vi "player.vi"() -> ()   [LabVIEW 2022 SP3]
uses:
  <vilib>/DAQmx/write.llb/DAQmx Write (Digital 1D Bool 1Chan 1Samp).vi
  <vilib>/DAQmx/create/channels.llb/DAQmx Create Channel (DO-Digital Output).vi
  <vilib>/Utility/file.llb/Read Delimited Spreadsheet (DBL).vi
  <vilib>/DAQmx/miscellaneous.llb/DAQmx Fill In Error Info.vi
panel:
  in  "Speed*X(If you want to play X times faster, enter X)":dbl=1.0
  in  "Backwards Mode (Forwards moves the light left to right, top to bottom)":bool
  in  "Choose LED Array (leftmost LED=top switch, rightmost LED=bottom switch":bool[](array[boolean])=[TRUE, FALSE, FALSE, FALSE, FALSE, FALSE, FALSE, FALSE]
  out "Numeric 3":dbl
  out "Numeric 2":dbl
  out "Last Wait":dbl
  out "Wait Times":dbl[](array[numeric])
  out "LEDs":bool[](array[boolean])
  out "error out":errorcluster
  in  "stop":bool
  # "LED Player! Play your own Christmas pattern!"
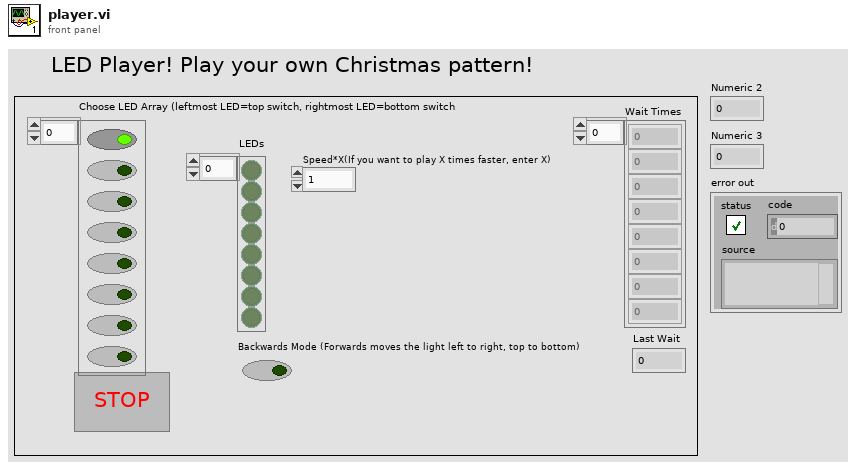
[diagram p1: front panel]
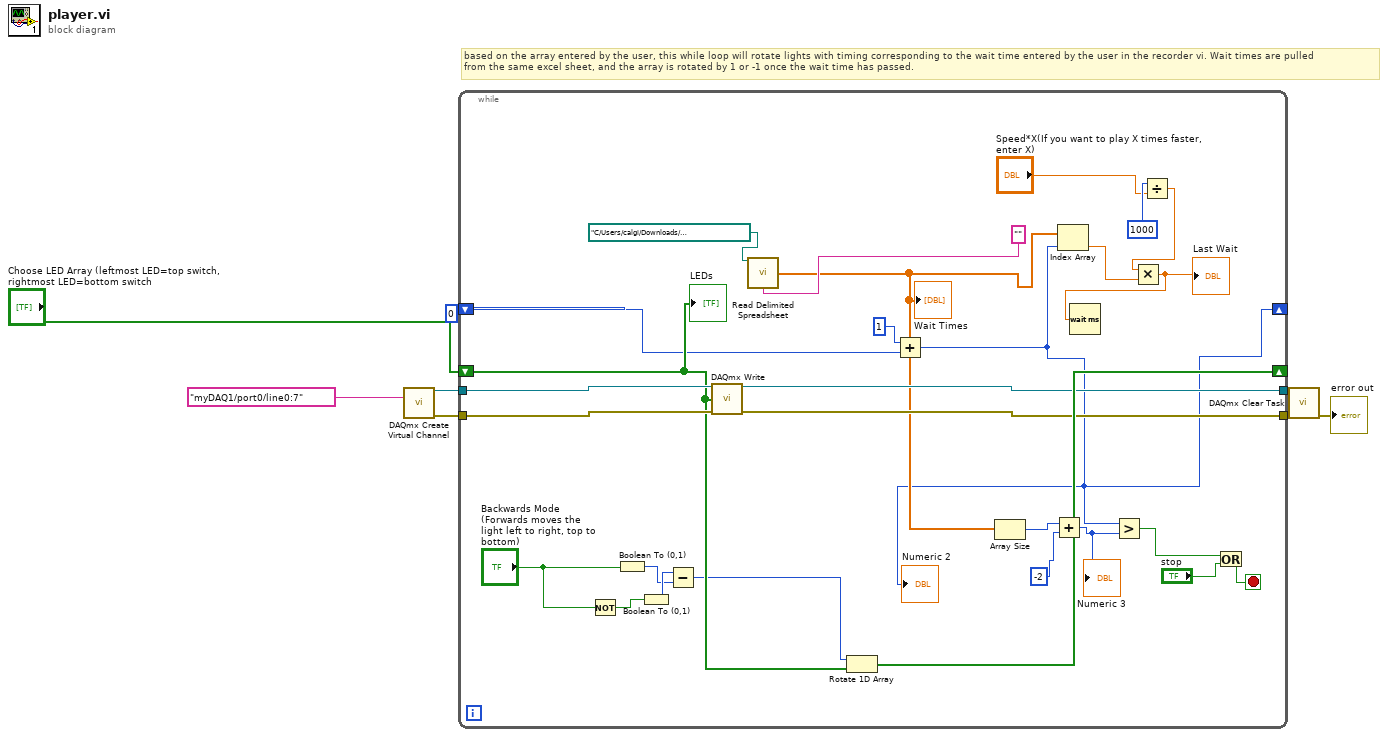
[diagram p0: block diagram]
diagram:
  # "based on the array entered by the user, this while loop will rotate lights with timing corresponding to the wait time entered by the user in the recorder vi. Wait times are pulled\nfrom the same excel sheet, and the array is rotated by 1 or -1 once the wait time has passed."
  n1 = call-poly <vilib>:"DAQmx Create Virtual Channel.vi"("lines"=tag "myDAQ1/port0/line0:7") -> ("task out"=w7:refnum<k21>, "error out"=w6:errorcluster)  [unwired: 13 in]
  n2 = while {
    shift-right: [w36] -> _
    shift-left: "Choose LED Array (leftmost LED=top switch, rightmost LED=bottom switch" -> [w31]
    tunnel: w7 -> [w35]
    tunnel: w6 -> [w34]
    tunnel: [w33] -> w5
    tunnel: [w32] -> w4
    shift-right: [w19] -> _
    shift-left: 0 -> [w28]
    stop <- w20 stop-if-true
    n3 = Not(x="Backwards Mode (Forwards moves the light left to right, top to bottom)") -> (.not. x?=w17:bool)
    n4 = Boolean To (0,1)(Boolean="Backwards Mode (Forwards moves the light left to right, top to bottom)") -> (0, 1=w14:i16)
    n5 = Boolean To (0,1)(Boolean=w17) -> (0, 1=w15:i16)
    n6 = Subtract(x=w15, y=w14) -> (x-y=w13:i16)
    n7 = call-poly <vilib>:"DAQmx Write.vi"("task/channels in"=w35, "data"=w31, "error in"=w34) -> ("task out"=w33:refnum<k21>, "error out"=w32:errorcluster)  [unwired: 10 in, 1 out]
    n8 = call-poly <vilib>:"Read Delimited Spreadsheet.vi"("file path (dialog if empty)"=path "C:/Users/calgi/Downloads/keyboardpatternBeta.csv", "delimiter (\\t)"="") -> ("first row"=w25:dbl[])  [unwired: 8 in, 5 out]
    "Wait Times" <- w25
    n9 = Rotate 1D Array(1:w31, 2:w13) -> (0:w36:bool[])
    n10 = Add(x=1, y=w28) -> (x+y=w19:i32)
    "Numeric 2" <- w19
    n11 = Array Size(array=w25) -> (size(s)=w24:i32)
    n12 = Add(x=w24, y=-2) -> (x+y=w18:i32)
    "Numeric 3" <- w18
    n13 = Index Array(array=w25, index=w19) -> (element=w30:dbl)
    n14 = Greater?(x=w19, y=w18) -> (0:w21:bool)
    n15 = Divide(x=1000, y="Speed*X(If you want to play X times faster, enter X)") -> (x/y=w9:dbl)
    n16 = Multiply(x=w9, y=w30) -> (x*y=w26:dbl)
    "Last Wait" <- w26
    n17 = Wait (ms)(milliseconds to wait=w26) -> ()  [unwired: 1 out]
    n18 = Or(x=w21, y="stop") -> (x .or. y?=w20:bool)
    "LEDs" <- w31
  }
  n19 = call <vilib>:"DAQmx Clear Task.vi"("task in"=w5, "error in"=w4) -> ("error out"=→"error out":errorcluster)  [unwired: 13 in]
